vi "Close Channel.vi"(8 "error in (no error)":errorcluster, 11 "Topic  (ALL)":string="*") -> (0 "error out":errorcluster)   [LabVIEW 2020, in "Actor Pub Sub Channels.lvlib"]
uses:
  Actor Pub Sub Channels.lvlib
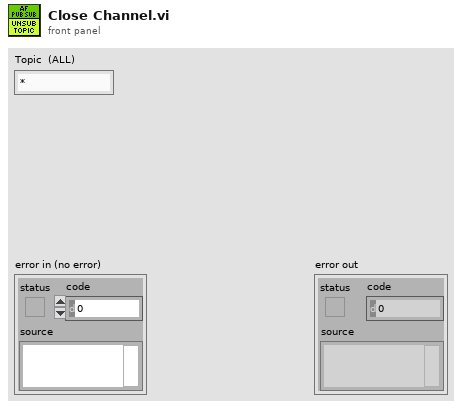
[diagram p1: front panel]
types:
  T1 = enum16{"Nothing", "Get Channel", "Get Or Create Channel", "Close Channel", "Dispose"}
  T2 = map{string, refnum<class "Pub Sub Message Channel.lvclass">}
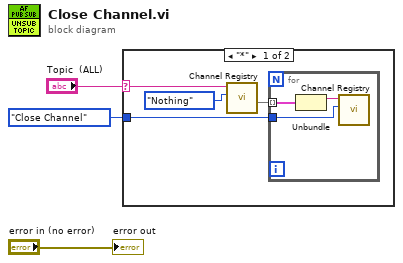
[diagram p0: block diagram]
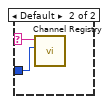
[diagram p2: hidden frame]
diagram:
  n1 = case shown="\"*\"" "Topic  (ALL)" {
    selector: "Topic  (ALL)" -> [w6 w11]
    tunnel: T1."Close Channel" ("Action") -> [w4 w12]
    frame "*" {
      n2 = call "Channel Registry.vi"("Action"=T1."Nothing", "Topic"=w6) -> ("Registered Channels"=w5:T2)  [unwired: 7 in, 2 out]
      n3 = for {
        tunnel: w5 -> [w10] mode=indexing
        tunnel: w4 -> [w9]
        n4 = Unbundle(w10) -> ("Topic"=w8:string)  [unwired: 1 out]
        n5 = call "Channel Registry.vi"("Action"=w9, "Topic"=w8) -> ()  [unwired: 7 in, 3 out]
      }
    }
    frame Default {
      n6 = call "Channel Registry.vi"("Action"=w12, "Topic"=w11) -> ()  [unwired: 7 in, 3 out]
    }
  }
  "error out" <- "error in (no error)"
